vi "move_shoot_collect.vi"(8 "Slot 4":bool=TRUE, 9 "Slot 3":bool=TRUE, 10 "Slot 2":bool, 11 "Slot 1":bool) -> (0 "Move up 4":bool, 1 "Move Up 3":bool, 2 "Move Up 2":bool, 3 "Shoot":bool, 4 "Collect":bool)   [LabVIEW 2012]
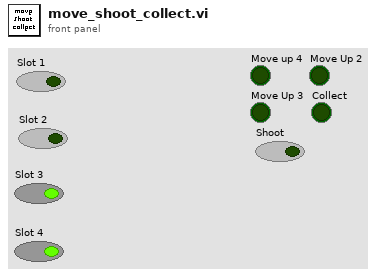
[diagram p1: front panel]
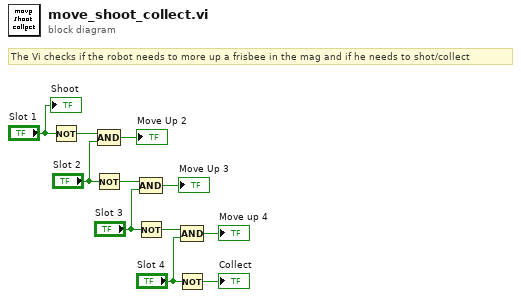
[diagram p0: block diagram]
diagram:
  # "The Vi checks if the robot needs to more up a frisbee in the mag and if he needs to shot/collect"
  n1 = Not(x="Slot 1") -> (.not. x?=w6:bool)
  n2 = Not(x="Slot 2") -> (.not. x?=w8:bool)
  n3 = Compound Arithmetic op=AND(w6, "Slot 2") -> (→"Move Up 2":bool)
  n4 = Not(x="Slot 3") -> (.not. x?=w10:bool)
  n5 = Compound Arithmetic op=AND(w8, "Slot 3") -> (→"Move Up 3":bool)
  n6 = Not(x="Slot 4") -> (.not. x?=→"Collect":bool)
  n7 = Compound Arithmetic op=AND(w10, "Slot 4") -> (→"Move up 4":bool)
  "Shoot" <- "Slot 1"
